vi "led_initallchannels.vi"(8 "ERROR":errorcluster, 11 "Channels":i32) -> (0 "ERROR OUT":errorcluster, 3 "Device Handle Out":u32)   [LabVIEW 2013]
panel:
  out "SerialNumber":string
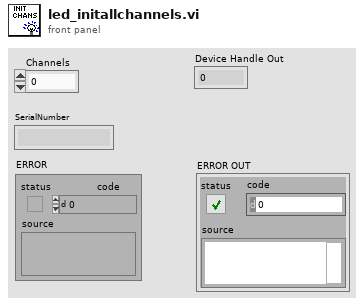
[diagram p1: front panel]
types:
  T1 = enum16{"Set Mode", "Set Normal Current ", "Set Strobe Parameters", "Set Normal Parameters", "Set Strobe Profile "}
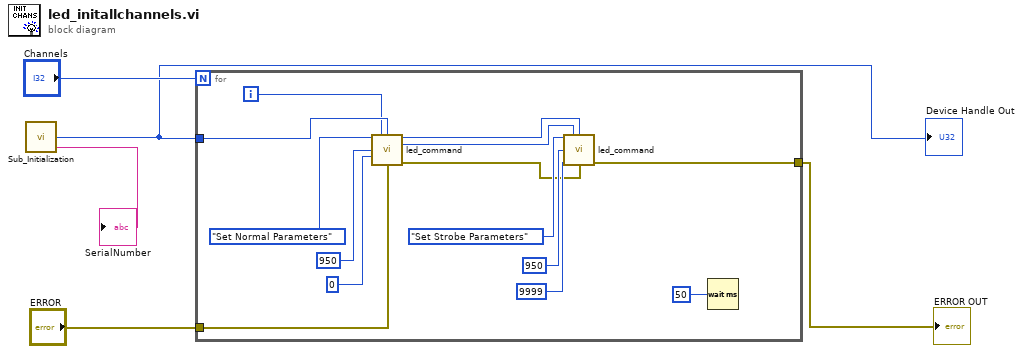
[diagram p0: block diagram]
diagram:
  n1 = call "Sub_Initialization.vi"() -> ("SerialNumber"=→"SerialNumber":string, "DeviceHandle"=w2:u32)  [unwired: 1 out]
  "Device Handle Out" <- w2
  n2 = for {
    N: "Channels" -> [_]
    tunnel: w2 -> [w16]
    tunnel: "ERROR" -> [w11]
    tunnel: [w6] -> w1
    i -> [w7]
    n3 = call "led_command.vi"("COMMAND"=T1."Set Normal Parameters", "Channel"=w7, "Device Handle"=w16, "Imax"=u32 950, "Iset"=u32 0, "ERROR"=w11) -> ("Device Handle Out"=w15:u32, "Channel Out"=w14:i32, "ERROR OUT"=w8:errorcluster)  [unwired: 6 in, 1 out]
    n4 = call "led_command.vi"("COMMAND"=T1."Set Strobe Parameters", "Channel"=w14, "Device Handle"=w15, "Imax"=u32 950, "Repeats"=u32 9999, "ERROR"=w8) -> ("ERROR OUT"=w6:errorcluster)  [unwired: 6 in, 3 out]
    n5 = Wait (ms)(milliseconds to wait=u32 50) -> ()  [unwired: 1 out]
  }
  "ERROR OUT" <- w1
